vi "Ex5 Threshold.vi"() -> ()   [LabVIEW 2020]
panel:
  in  "Range (Threshold 1)":cluster{"Lower value":sgl, "Upper value":sgl}={"Lower value"=129.0, "Upper value"=255.0}
  out "Color Channel":T1(plugin-control)
  out "Image":T1(plugin-control)
  out "error out":errorcluster
  in  "File Path":path
  # "EX.5 THRESHOLD"
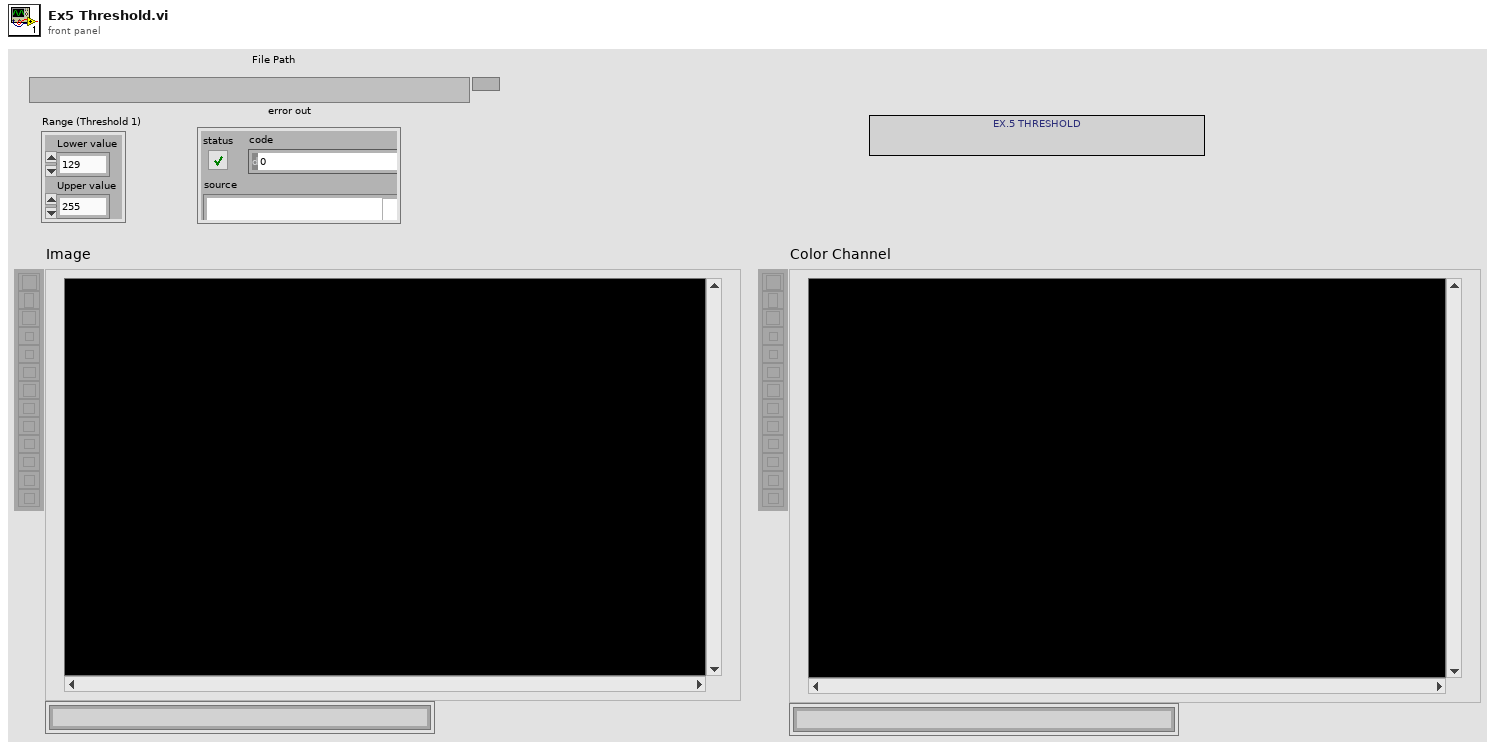
[diagram p1: front panel]
types:
  T1 = typedef "IMAQ Image.ctl" = refnum<image>
  T2 = typedef "Image Type" = u32
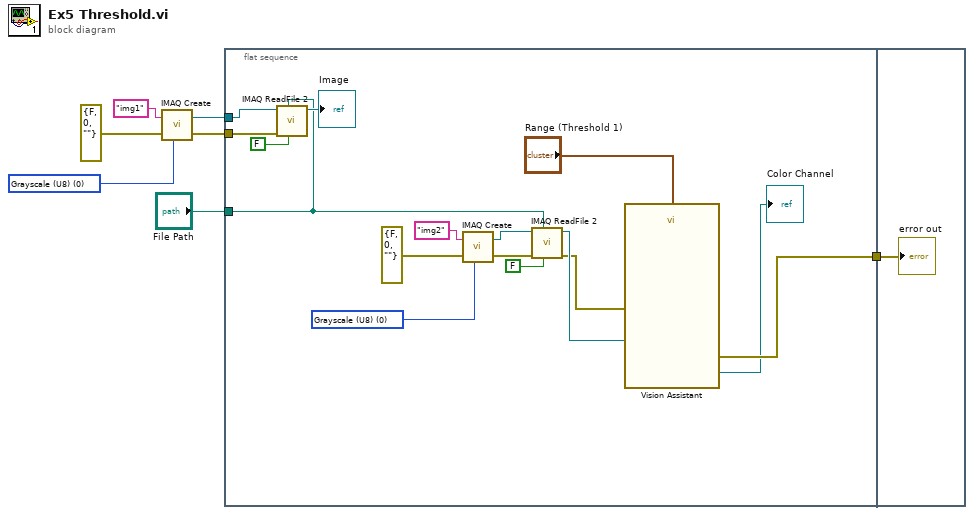
[diagram p0: block diagram]
diagram:
  w2 = T2 0 items=["Grayscale (U8)", "Grayscale (I16)", "Grayscale (SGL)", "Complex (CSG)", "RGB (U32)", "HSL (U32)", "RGB (U64)", "Grayscale (U16)"] ("Image Type")
  n1 = call "IMAQ Create"("Image Name"="img1", "Image Type"=w2, "error in (no error)"=errorcluster {"status"=FALSE, "code"=0, "source"=""}) -> ("New Image"=w3:T1, "error out"=w4:errorcluster)  [unwired: 2 in]
  n2 = flat-sequence {
    tunnel: "File Path" -> [w12]
    tunnel: w4 -> [w22]
    tunnel: w3 -> [w21]
    tunnel: [w19] -> w1
    tunnel: w1 -> [w24]
    frame #0 {
      w16 = T2 0 items=["Grayscale (U8)", "Grayscale (I16)", "Grayscale (SGL)", "Complex (CSG)", "RGB (U32)", "HSL (U32)", "RGB (U64)", "Grayscale (U16)"] ("Image Type")
      n3 = call "IMAQ ReadFile 2"("Use File Path Image Type"=FALSE, "File Path"=w12, "error in (no error)"=w22, "Image"=w21) -> ("Image Out"=→"Image":T1)  [unwired: 3 in, 4 out]
      n4 = call "IMAQ Create"("Image Name"="img2", "Image Type"=w16, "error in (no error)"=errorcluster {"status"=FALSE, "code"=0, "source"=""}) -> ("New Image"=w15:T1, "error out"=w14:errorcluster)  [unwired: 2 in]
      n5 = call "IMAQ ReadFile 2"("Use File Path Image Type"=FALSE, "File Path"=w12, "error in (no error)"=w14, "Image"=w15) -> ("error out"=w10:errorcluster, "Image Out"=w11:T1)  [unwired: 3 in, 3 out]
      n6 = call "Vision Assistant"("Image In"=w11, "Range (Threshold 1)"="Range (Threshold 1)", "error in"=w10) -> ("Image Out"=→"Color Channel":T1, "error out"=w19:errorcluster)  [unwired: 23 in]
    }
    frame #1 {
      "error out" <- w24
    }
  }
